vi "Velocity_Calc.vi"(6 "Velocity in":dbl, 8 "Last time in":dbl, 9 "Time":dbl, 10 "Last acceleration in":dbl, 11 "Acceleration":dbl) -> (0 "Last time out":dbl, 3 "Last acceleration out":dbl, 4 "Velocity out":dbl)   [LabVIEW 2017]
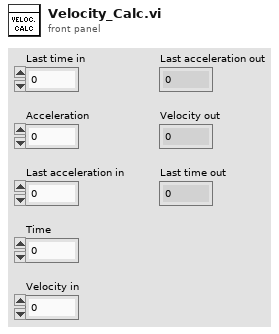
[diagram p1: front panel]
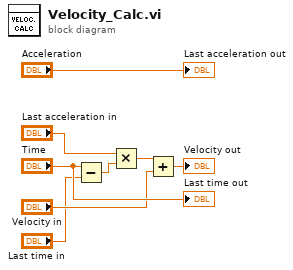
[diagram p0: block diagram]
diagram:
  n1 = Subtract(x="Time", y="Last time in") -> (x-y=w2:dbl)
  n2 = Multiply(x="Last acceleration in", y=w2) -> (x*y=w5:dbl)
  n3 = Add(x=w5, y="Velocity in") -> (x+y=→"Velocity out":dbl)
  "Last time out" <- "Time"
  "Last acceleration out" <- "Acceleration"
